vi "Character Tester.vi"() -> ()   [LabVIEW 2015]
uses:
  REV Robotics Digit - Library.llb/REVDigit.lvlib
panel:
  out "Character Output":u16 format="0b%016b"
  in  "14":bool
  in  "13":bool
  in  "12":bool
  in  "11":bool
  in  "10":bool
  in  "9":bool
  in  "8":bool
  in  "7":bool
  in  "6":bool
  in  "5":bool
  in  "4":bool
  in  "3":bool
  in  "2":bool
  in  "1":bool
  in  "0":bool
  in  "ASCII":u8
  in  "stop":bool
  out "Character":string
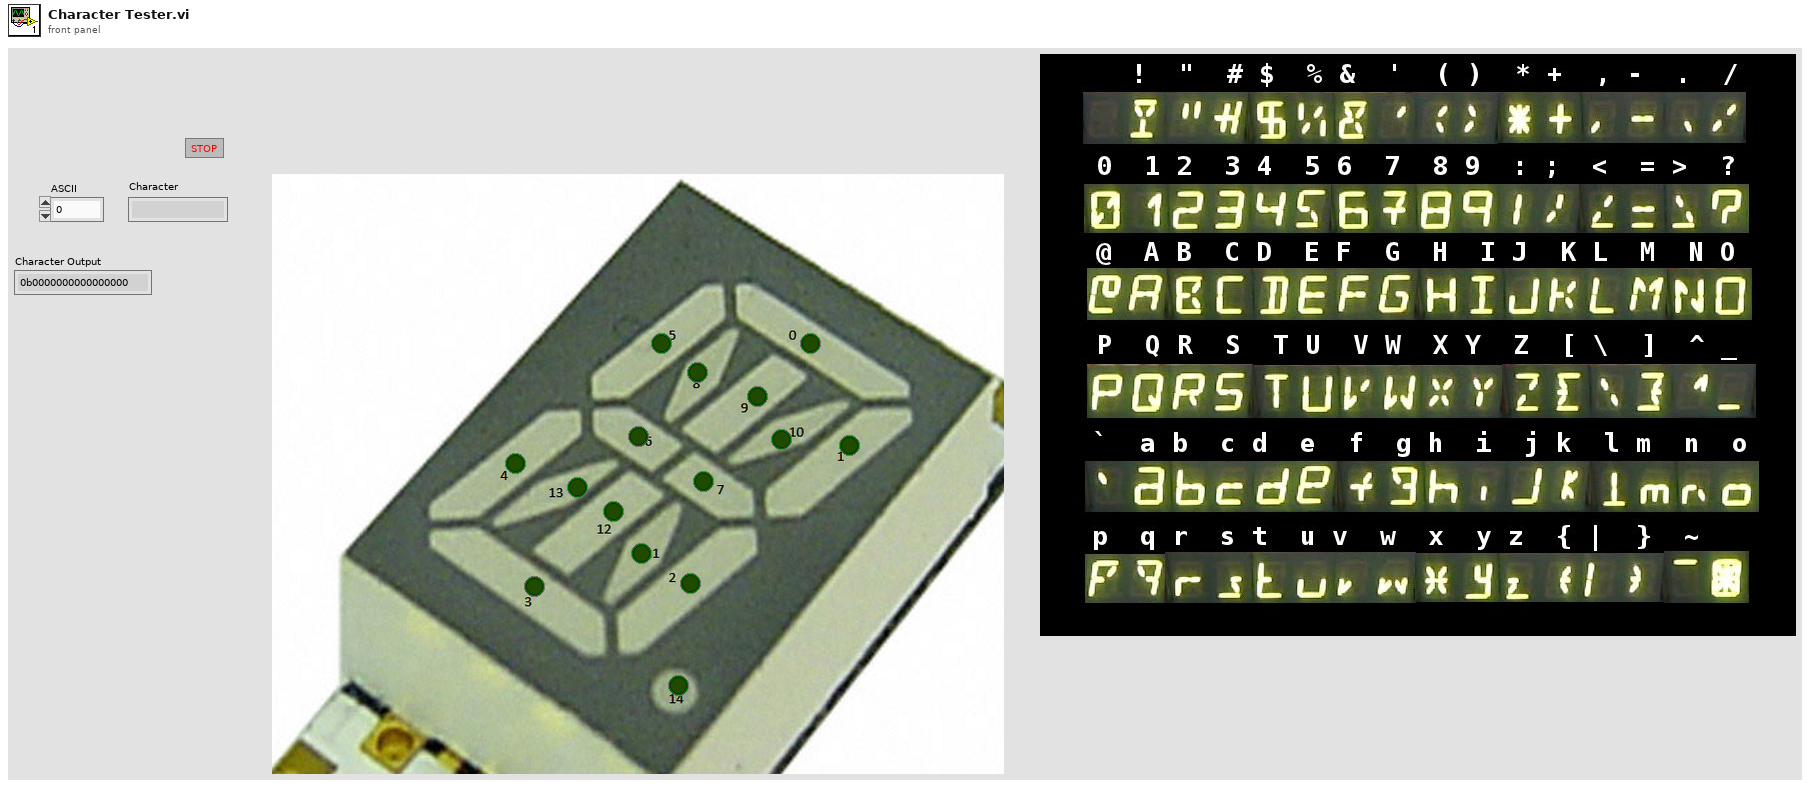
[diagram p1: front panel]
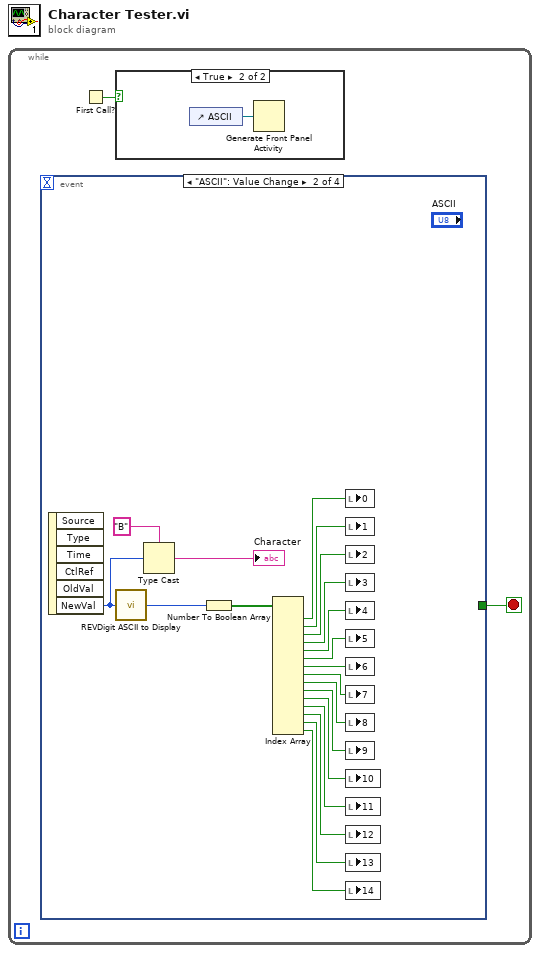
[diagram p0: block diagram]
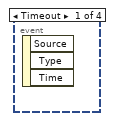
[diagram p3: hidden frame]
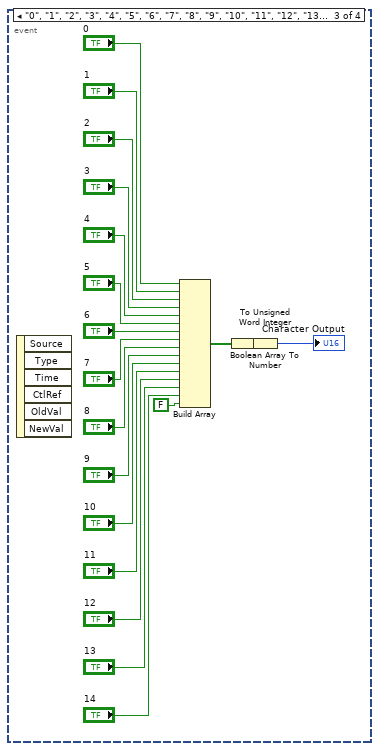
[diagram p4: hidden frame]
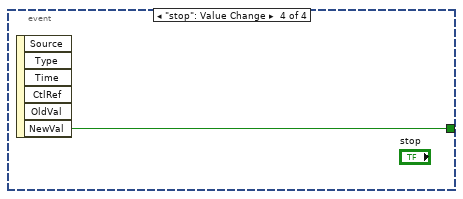
[diagram p5: hidden frame]
diagram:
  n1 = while {
    stop <- w2 stop-if-true
    n2 = event shown="[1] \"ASCII\": Value Change" {
      selector: _ -> [_ _ _ _]
      dyn-events: _ -> [_ _ _ _]
      timeout: _ -> [_ _ _ _]
      tunnel: [_ _ _ w43] -> w2
      event Timeout {
        n3 = event-data() -> ()  [unwired: 1 in, 3 out]
      }
      event "ASCII": Value Change {
        n4 = event-data() -> ("NewVal"=w19:u8)  [unwired: 1 in, 5 out]
        n5 = call "REVDigit ASCII to Display.vi"("ASCII Value"=w19) -> ("Digit Character Value"=w23:u16)
        n6 = Type Cast(type="B" ("Character"), x=w19) -> (*(type *) &x=→"Character":string)
        n7 = Number To Boolean Array(number=w23) -> (Boolean array=w22:bool[])
        n8 = Index Array(array=w22) -> (element #1=w18:bool, element #2=w17:bool, element #3=w16:bool, element #4=w15:bool, element #5=w14:bool, element #6=w13:bool, element #7=w12:bool, element #8=w11:bool, element #9=w10:bool, element #10=w9:bool, element #11=w8:bool, element #12=w7:bool, element #13=w6:bool, element #14=w5:bool, element #15=w4:bool)  [unwired: 15 in]
        n9 = local write "0"(w18) -> ()
        n10 = local write "1"(w17) -> ()
        n11 = local write "2"(w16) -> ()
        n12 = local write "3"(w15) -> ()
        n13 = local write "4"(w14) -> ()
        n14 = local write "5"(w13) -> ()
        n15 = local write "6"(w12) -> ()
        n16 = local write "7"(w11) -> ()
        n17 = local write "8"(w10) -> ()
        n18 = local write "9"(w9) -> ()
        n19 = local write "10"(w8) -> ()
        n20 = local write "11"(w7) -> ()
        n21 = local write "12"(w6) -> ()
        n22 = local write "13"(w5) -> ()
        n23 = local write "14"(w4) -> ()
      }
      event "0", "1", "2", "3", "4", "5", "6", "7", "8", "9", "10", "11", "12", "13", "14": Value Change {
        n24 = event-data() -> ()  [unwired: 1 in, 6 out]
        n25 = Build Array("0", "1", "2", "3", "4", "5", "6", "7", "8", "9", "10", "11", "12", "13", "14", FALSE ("element")) -> (w26:bool[])
        n26 = Boolean Array To Number(Boolean array=w26) -> (number=w25:u32)
        n27 = To Unsigned Word Integer(number=w25) -> (unsigned 16bit integer=→"Character Output":u16)
      }
      event "stop": Value Change {
        n28 = event-data() -> ("NewVal"=w43:bool)  [unwired: 1 in, 5 out]
      }
    }
    n29 = First Call?() -> (First Call?: T/F=w1:bool)
    n30 = case shown="True" w1 {
      frame False {
      }
      frame True {
        n31 = control-ref of="ASCII"() -> (w3:refnum<vi>)
        n32 = Generate Front Panel Activity(w3) -> ()
      }
    }
  }
